vi "Climber_Teleop.vi"(1 "Joystick_Out":T1) -> ()   [LabVIEW 2020]
uses:
  Utility VIs/Joystick_Controls.ctl
  Subsystems/Climber/Climber_Cluster.ctl
  Subsystems/Climber/Climber_Control_States.ctl
  Globals/Climber_Globals.vi
panel:
  in  "Inner Pivot Left Trigger Deadzone Size":dbl=0.1 format="%#_13g"
  in  "Inner Pivot Right Trigger Deadzone Size":dbl=0.1 format="%#_13g"
  in  "Outer Elevator Deadzone Size":dbl=0.1 format="%#_13g"
  in  "Outer Pivot Deadzone Size":dbl=0.1 format="%#_13g"
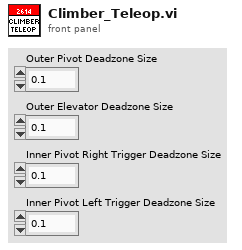
[diagram p1: front panel]
types:
  T1 = typedef "Joystick_Controls.ctl" = cluster{"Pilot Left Joystick X":dbl, "Pilot Left Joystick Y":dbl, "Pilot A Button":bool, "Pilot B Button":bool, "Pilot X Button":bool, "Pilot Y Button":bool, "Pilot Left Bumper":bool, "Pilot Right Bumper":bool, "Pilot View Button":bool, "Pilot Menu Button":bool, "Pilot Left Joystick Press":bool, "Pilot Right Joystick Press":bool, "Pilot Left Trigger":dbl, "Pilot Right Joystick X":dbl, "Pilot Right Joystick Y":dbl, "Pilot Right Trigger":dbl, "Copilot Left Joystick X":dbl, "Copilot Left Joystick Y":dbl, "Copilot A Button":bool, "Copilot B Button":bool, "Copilot X Button":bool, "Copilot Y Button":bool, "Copilot Left Bumper":bool, "Copilot Right Bumper":bool, "Copilot View Button":bool, "Copilot Menu Button":bool, "Copilot Left Joystick Press":bool, "Copilot Right Joystick Press":bool, "Copilot Left Trigger":dbl, "Copilot Right Joystick X":dbl, "Copilot Right Joystick Y":dbl, "Copilot Right Trigger":dbl, "Pilot D-pad North":bool, "Pilot D-pad South":bool, "Pilot D-pad East":bool, "Pilot D-pad West":bool, "Pilot D-pad NE ":bool, "Pilot D-pad SE":bool, "Pilot D-pad SW":bool, "Pilot D-pad NW":bool, "CoPilot D-pad North":bool, "CoPilot D-pad South":bool, "CoPilot D-pad East":bool, "CoPilot D-pad West":bool, "CoPilot D-pad NE":bool, "CoPilot D-pad SE":bool, "CoPilot D-pad SW":bool, "CoPilot D-pad NW":bool, "Pilot Left Trigger Pressed":bool, "Pilot Right Trigger Pressed":bool, "CoPilot Left Trigger Pressed":bool, "CoPilot Right Trigger Pressed":bool}
  T2 = typedef "Climber_Cluster.ctl" = cluster{"Control_State":T3, "Outer_Arm_Pivot_Throttle":dbl, "Outer_Arm_Elevator_Throttle":dbl, "Inner_Arm_Pivot_Throttle":dbl, "Enable_Climber_Sequence":bool}
  T3 = typedef "Climber_Control_States.ctl" = enum16{"No-Op", "Manual_%Vbus", "Correct_Outer_Pivot_Offset", "Climbing_Sequence", "Tune_PIDs"}
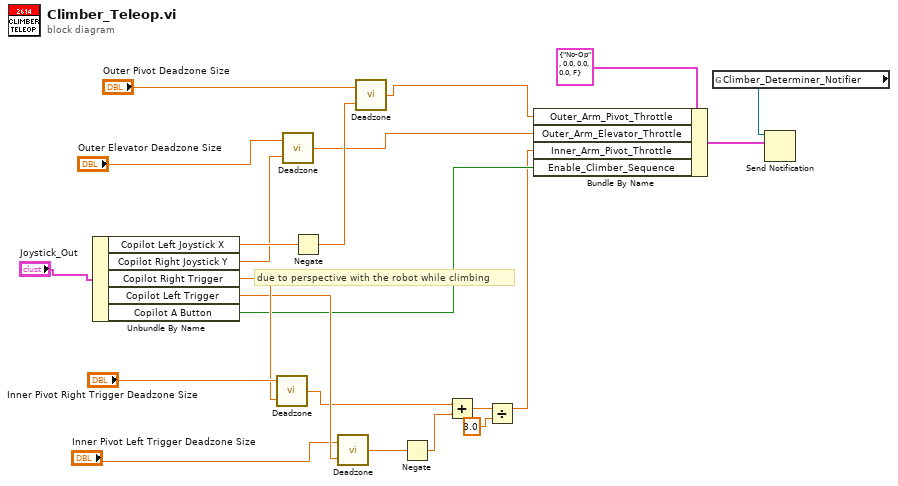
[diagram p0: block diagram]
diagram:
  # "due to perspective with the robot while climbing"
  n1 = Unbundle By Name("Joystick_Out") -> ("Copilot Left Joystick X"=w18:dbl, "Copilot Right Joystick Y"=w17:dbl, "Copilot Right Trigger"=w14:dbl, "Copilot Left Trigger"=w13:dbl, "Copilot A Button"=w4:bool)
  n2 = call "Deadzone.vi"("Joystick Value Input"=w14, "Deadzone Size"="Inner Pivot Right Trigger Deadzone Size") -> ("Corrected Joystick Value"=w6:dbl)  [unwired: 1 in]
  n3 = call "Deadzone.vi"("Joystick Value Input"=w17, "Deadzone Size"="Outer Elevator Deadzone Size") -> ("Corrected Joystick Value"=w7:dbl)  [unwired: 1 in]
  n4 = Negate(x=w18) -> (-x=w10:dbl)
  n5 = call "Deadzone.vi"("Joystick Value Input"=w13, "Deadzone Size"="Inner Pivot Left Trigger Deadzone Size") -> ("Corrected Joystick Value"=w11:dbl)  [unwired: 1 in]
  n6 = call "Deadzone.vi"("Joystick Value Input"=w10, "Deadzone Size"="Outer Pivot Deadzone Size") -> ("Corrected Joystick Value"=w8:dbl)  [unwired: 1 in]
  n7 = Negate(x=w11) -> (-x=w5:dbl)
  n8 = Add(x=w6, y=w5) -> (x+y=w2:dbl)
  n9 = Divide(x=w2, y=3.0) -> (x/y=w3:dbl)
  n10 = Bundle By Name(cluster=T2 {"Control_State"=enum."No-Op", "Outer_Arm_Pivot_Throttle"=0.0, "Outer_Arm_Elevator_Throttle"=0.0, "Inner_Arm_Pivot_Throttle"=0.0, "Enable_Climber_Sequence"=FALSE} ("Climber_Cluster"), "Outer_Arm_Pivot_Throttle"=w8, "Outer_Arm_Elevator_Throttle"=w7, "Inner_Arm_Pivot_Throttle"=w3, "Enable_Climber_Sequence"=w4) -> (w21:T2)
  n11 = global read "Climber_Globals.vi" "Climber_Determiner_Notifier"() -> (w22:refnum<notifier>)
  n12 = Send Notification(notification=w21, notifier=w22) -> ()  [unwired: 1 in, 2 out]
